vi "Session_Open.vi"(0 "Port Number":u16=1444, 1 "CCS Base Folder 2":path=path "C:/ti/ccs1020/ccs/ccs_base", 2 "CCXML File (target configuration)":path=path "D:/Projects/C2000/Grande/c2000_topogrande_avv/bitfield-submodule/common/targetConfigs/TMS320F280039C.ccxml", 3 "program file":path=path "D:/Projects/C2000/Grande/c2000_topogrande_avv/testcases_non_avv/ADC/adc_off-gain/Debug/topog_adc_off-gain.out", 5 "Core Number":u16=1, 11 "error in (no error)":errorcluster) -> (4 "Programed":bool=TRUE, 15 "error out":errorcluster)   [LabVIEW 2019]
uses:
  <userlib>/_TI-LA/Reusable/CCS/APIs/CCS.lvlib
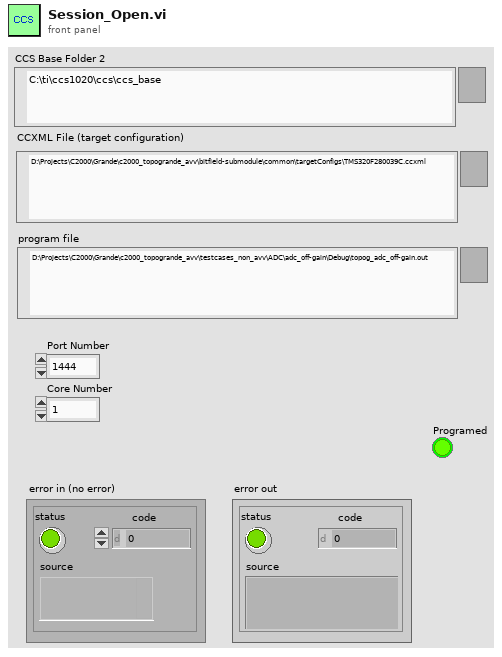
[diagram p1: front panel]
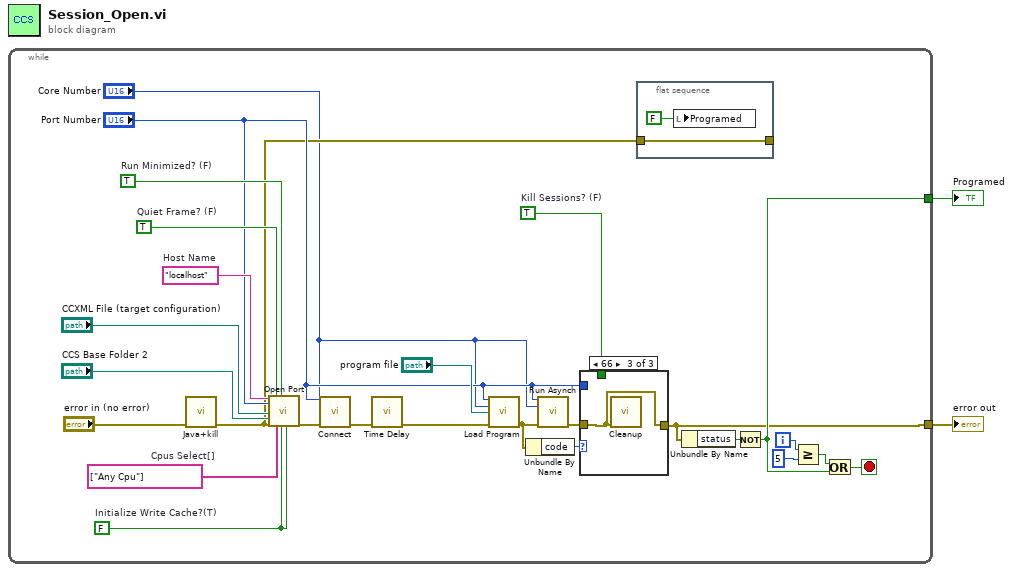
[diagram p0: block diagram]
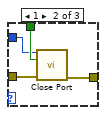
[diagram p3: hidden frame]
diagram:
  n1 = while {
    tunnel: [w8] -> w2
    tunnel: [w5] -> w1
    i -> [w6]
    stop <- w7 stop-if-true
    w12 = TRUE  # Kill Sessions? (F)
    w21 = FALSE  # Initialize Write Cache?(T)
    w22 = string[] ["Any Cpu"]  # Cpus Select[]
    w23 = TRUE  # Run Minimized? (F)
    w24 = TRUE  # Quiet Frame? (F)
    w27 = "localhost"  # Host Name
    n2 = call "Java+kill.vi"("error in (no error)"="error in (no error)") -> ("error out"=w9:errorcluster)  [unwired: 10 in]
    n3 = call <userlib>:"Open Port.vi"("Host Name"=w27, "Port Number"="Port Number", "CCXML File"="CCXML File (target configuration)", "CCS Base Folder"="CCS Base Folder 2", "error in"=w9, "Quiet Frame? (F)"=w24, "Cpus Select[]"=w22, "Run Minimized? (F)"=w23, "Initialize Write Cache?(T)"=w21, "Initialize Symbol Cache?(T)"=w21) -> ("error out"=w28:errorcluster)  [unwired: 7 in, 2 out]
    n4 = call <userlib>:"Connect.vi"("Port Number"="Port Number", "Core Number"="Core Number", "error in"=w28) -> ("error out"=w15:errorcluster)  [unwired: 10 in, 2 out]
    n5 = call "Time Delay"("error in (no error)"=w15) -> ("error out"=w3:errorcluster)  [unwired: 10 in]
    n6 = call <userlib>:"Load Program.vi"("Port Number"="Port Number", "Core Number"="Core Number", "Program File Path"="program file", "error in"=w3) -> ("error out"=w14:errorcluster)  [unwired: 7 in, 4 out]
    n7 = Unbundle By Name(w14) -> ("code"=w13:i32)
    n8 = call <userlib>:"Run Asynch.vi"("Port Number"="Port Number", "Core Number"="Core Number", "error in"=w14) -> ("error out"=w11:errorcluster)  [unwired: 10 in, 2 out]
    n9 = case shown="66" w13 {
      tunnel: w12 -> [_ w35 _]
      tunnel: w11 -> [w31 w34 w36]
      tunnel: [w31 w33 w36] -> w5
      tunnel: "Port Number" -> [_ w32 _]
      frame Default {
      }
      frame 1 {
        n10 = call <userlib>:"Close Port.vi"("Port Number"=w32, "Kill Sessions? (F)"=w35, "error in"=w34) -> ("error out"=w33:errorcluster)  [unwired: 10 in, 2 out]
      }
      frame 66 {
        n11 = call <userlib>:"Cleanup.vi"("error in"=w36) -> ()  [unwired: 14 in, 1 out]
      }
    }
    n12 = flat-sequence {
      tunnel: w9 -> [w29]
      tunnel: [w29] -> _
      frame #0 {
        n13 = local write "Programed"(FALSE ("Repeat")) -> ()
      }
    }
    n14 = Unbundle By Name(w5) -> ("status"=w17:bool)
    n15 = Not(x=w17) -> (.not. x?=w8:bool)
    n16 = Greater Or Equal?(x=w6, y=5) -> (x >= y?=w19:bool)
    n17 = Or(x=w19, y=w8) -> (x .or. y?=w7:bool)
  }
  "Programed" <- w2
  "error out" <- w1
